vi "Exercise 2 Solution.vi"() -> ()   [LabVIEW 2019]
panel:
  out "Random Value (0-1)":dbl format="%#_5g"
  out "Limit Exceeded?":bool
  in  "Limit (0-1)":dbl
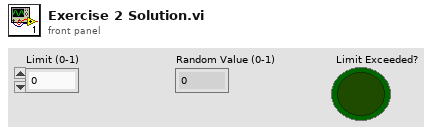
[diagram p1: front panel]
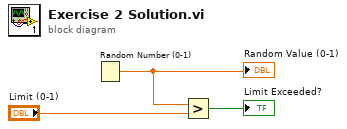
[diagram p0: block diagram]
diagram:
  n1 = Random Number (0-1)() -> (number: 0 to 1=w2:dbl)
  "Random Value (0-1)" <- w2
  n2 = Greater?(x=w2, y="Limit (0-1)") -> (0:→"Limit Exceeded?":bool)
